vi "Temperature Limit.vi"() -> ()   [LabVIEW 2015]
doc: "This VI simulates the acquisition of temperature, graphs the temperature, and notifies the user if the temperature is over the limit."
panel:
  in  "Start":bool
  in  "Delta t (ms)":i32(slide)=400 scale=50.0..500.0
  in  "Stop":bool
  in  "High Limit":dbl=28.0 format="%.2f"
  out "Temperature":cluster{"Temperature":dbl, "High Limit":dbl}(graph)={"Temperature"=85.88749999999999, "High Limit"=80.0}
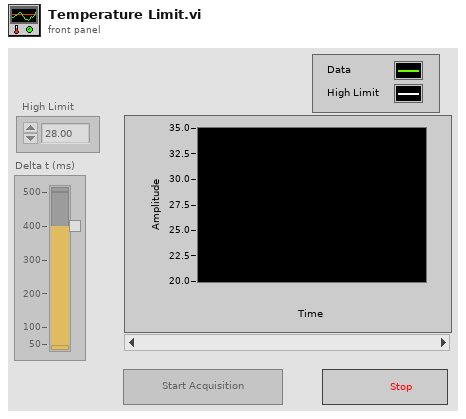
[diagram p1: front panel]
types:
  T1 = enum8{"Enabled", "Disabled", "Disabled and Grayed Out"}
  T2 = cluster{"Temperature Value":dbl, "High Limit":dbl}
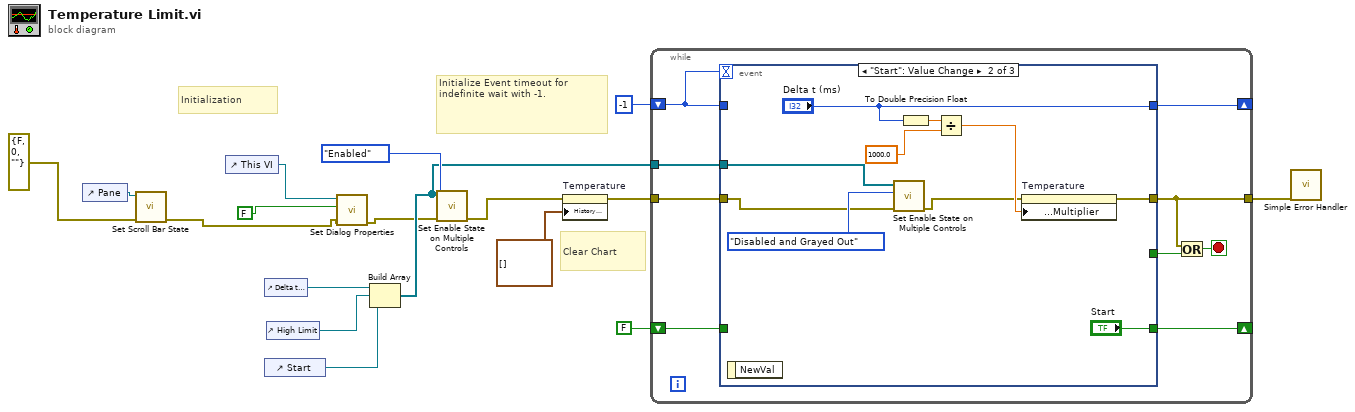
[diagram p0: block diagram]
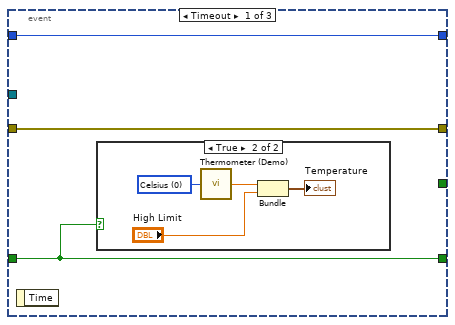
[diagram p2: hidden frame]
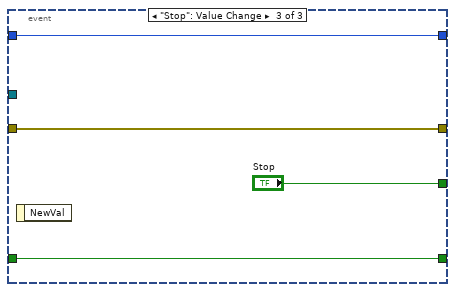
[diagram p4: hidden frame]
diagram:
  # "Clear Chart"
  # "Initialize Event timeout for indefinite wait with -1."
  # "Initialization"
  n1 = control-ref of="Pane"() -> (w9:refnum<vi>)
  n2 = call "Set Scroll Bar State.vi"("error in (no error)"=errorcluster {"status"=FALSE, "code"=0, "source"=""}, "Pane in"=w9) -> ("error out"=w2:errorcluster)  [unwired: 8 in, 1 out]
  n3 = control-ref of="This VI"() -> (w11:refnum<vi>)
  n4 = control-ref of="Delta t (ms)"() -> (w6:refnum<vi>)
  n5 = control-ref of="Start"() -> (w4:refnum<vi>)
  n6 = control-ref of="High Limit"() -> (w5:refnum<vi>)
  n7 = call "Set Dialog Properties.vi"("error in (no error)"=w2, "Boolean"=FALSE, "VI in"=w11) -> ("error out"=w1:errorcluster)  [unwired: 7 in, 1 out]
  n8 = Build Array(w6, w5, w4) -> (w3:refnum<vi>[])
  n9 = call "Set Enable State on Multiple Controls.vi"("Error In"=w1, "Disabled State"=T1."Enabled", "Controls"=w3) -> ("Error Out"=w8:errorcluster)  [unwired: 8 in]
  n10 = property on="Temperature" class="WFChart (strict)"(error in=w8, "History Data"=cluster{"Temperature":dbl, "High Limit":dbl}[] []) -> (error out=w16:errorcluster)  [unwired: 1 in, 1 out]
  n11 = while {
    tunnel: w16 -> [w26]
    tunnel: [w24] -> w14
    shift-right: [w22] -> _
    shift-left: FALSE ("Start") -> [w21]
    shift-right: [w20] -> _
    shift-left: -1 ("Delta t (ms)") -> [w19]
    tunnel: w3 -> [w18]
    stop <- w25 stop-if-true
    n12 = event shown="[1] \"Start\": Value Change" {
      selector: _ -> [_ _ _]
      dyn-events: _ -> [_ _ _]
      timeout: w19 -> [_ _ _]
      tunnel: [_ _ "Stop"] -> w23
      tunnel: w26 -> [w29 w35 w46]
      tunnel: [w29 w43 w46] -> w24
      tunnel: [w27 "Start" w45] -> w22
      tunnel: w21 -> [w27 _ w45]
      tunnel: [w28 "Delta t (ms)" w44] -> w20
      tunnel: w19 -> [w28 _ w44]
      tunnel: w18 -> [_ w37 _]
      event Timeout {
        n13 = event-data() -> ()  [unwired: 1 in, 1 out]
        n14 = case shown="True" w27 {
          frame False {
          }
          frame True {
            w30 = u16 0 items=["Celsius", "Fahrenheit"] ("Units (0: Celsius)")
            n15 = call "Thermometer (Demo).vi"("Units (0: Celsius)"=w30) -> ("Temperature Value"=w31:dbl)
            n16 = Bundle("Temperature Value"=w31, "High Limit"="High Limit") -> (→"Temperature":T2)  [unwired: 1 in]
          }
        }
      }
      event "Start": Value Change {
        n17 = event-data() -> ()  [unwired: 1 in, 1 out]
        n18 = call "Set Enable State on Multiple Controls.vi"("Error In"=w35, "Disabled State"=T1."Disabled and Grayed Out", "Controls"=w37) -> ("Error Out"=w34:errorcluster)  [unwired: 8 in]
        n19 = To Double Precision Float(number="Delta t (ms)") -> (double precision float=w42:dbl)
        n20 = Divide(x=w42, y=1000.0) -> (x/y=w40:dbl)
        n21 = property on="Temperature" class="WFChart (strict)"(error in=w34, "X Scale.Offset and Multiplier:Multiplier"=w40) -> (error out=w43:errorcluster)  [unwired: 1 in, 1 out]
      }
      event "Stop": Value Change {
        n22 = event-data() -> ()  [unwired: 1 in, 1 out]
      }
    }
    n23 = Or(x=w24, y=w23) -> (x .or. y?=w25:bool)
  }
  n24 = call <vilib>:"Simple Error Handler.vi"("error in (no error)"=w14) -> ()  [unwired: 4 in, 5 out]
